vi "fgv_vision-info.vi"(7 "cmd":enum16{"read", "write"}(ring), 11 "image info":T1 {"Threshold Range"."Lower value" format="%#_3f"; "Threshold Range"."Upper value" format="%#_3g"}) -> (3 "image info out":T1 {"Threshold Range"."Lower value" format="%#_3f"; "Threshold Range"."Upper value" format="%#_3g"})   [LabVIEW 2019]
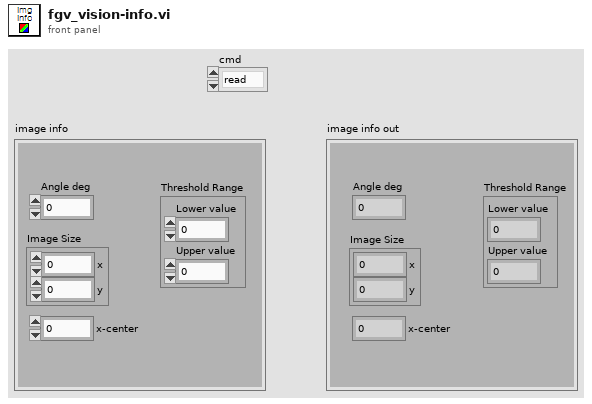
[diagram p1: front panel]
types:
  T1 = cluster{"x-center":dbl, "Image Size":cluster{"x":i32, "y":i32}, "Angle deg":sgl, "Threshold Range":cluster{"Lower value":sgl, "Upper value":sgl}}
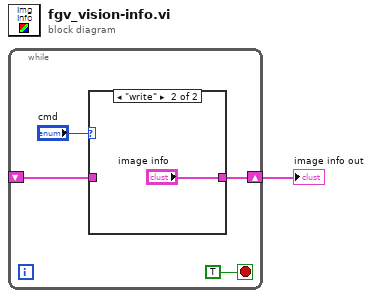
[diagram p0: block diagram]
diagram:
  n1 = while {
    shift-right: [w3] -> w1
    shift-left: _ -> [w2]
    stop <- TRUE stop-if-true
    n2 = case shown="\"write\"" "cmd" {
      tunnel: [w6 "image info"] -> w3
      tunnel: w2 -> [w6 _]
      frame "read", Default {
      }
      frame "write" {
      }
    }
  }
  "image info out" <- w1
